vi "statusQuery.vi"(8 "Reply size":i32, 11 "Device ID":i32) -> (0 "statusText":string, 3 "statusCode":i32)   [LabVIEW 2011]
panel:
  out "cyclic status":bool
  out "ramp status":bool
  out "ramp status 2":bool
  out "Reply":string
  out "frameStatus 2":bool
  out "unsigned byte array":u8[](array[numeric])
  out "1 min":u8
  out "1 max":u8
  out "2 min":u8
  out "2 max":u8
  out "frameStatus":bool
  out "Boolean array":bool[](array[boolean])
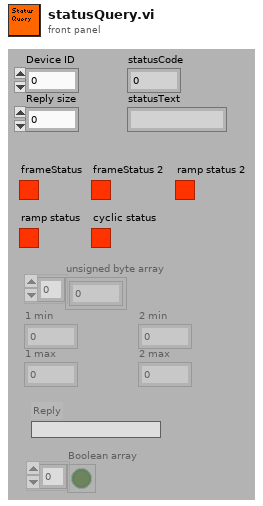
[diagram p1: front panel]
types:
  T1 = cluster{"unsigned byte array[0]":u8, "unsigned byte array[1]":u8, "unsigned byte array[2]":u8, "unsigned byte array[3]":u8, "unsigned byte array[4]":u8, "unsigned byte array[5]":u8, "unsigned byte array[6]":u8, "unsigned byte array[7]":u8, "unsigned byte array[8]":u8}
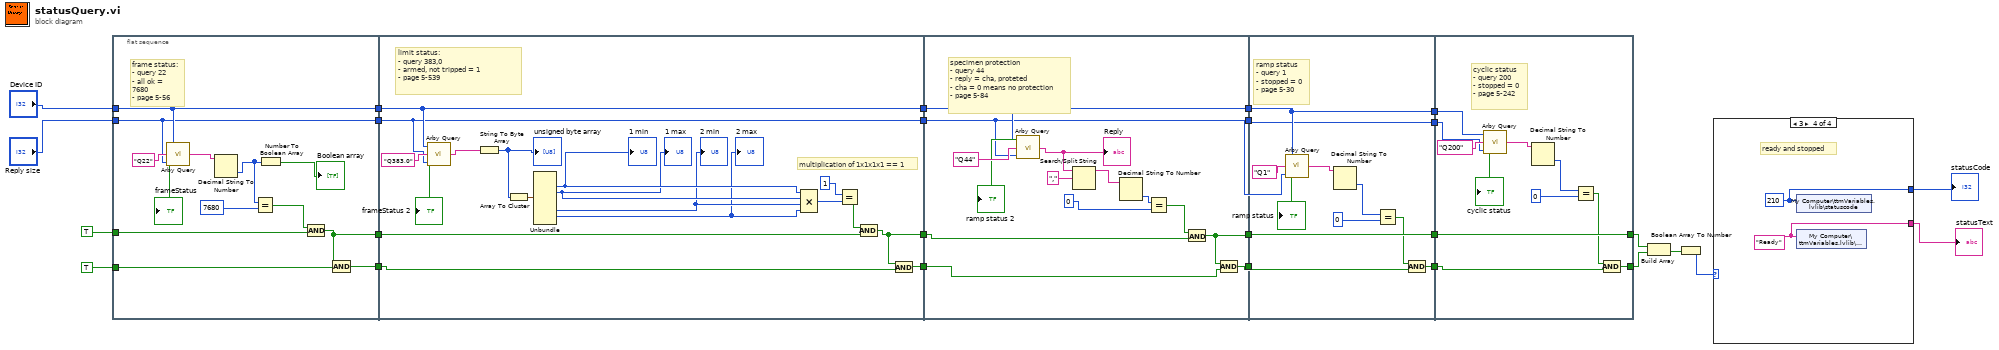
[diagram p0: block diagram]
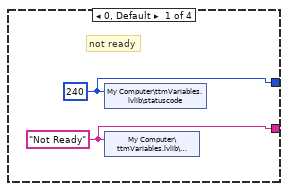
[diagram p2: hidden frame]
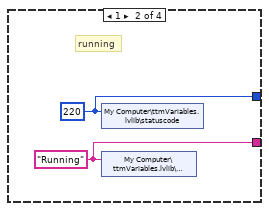
[diagram p3: hidden frame]
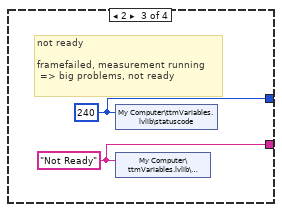
[diagram p4: hidden frame]
diagram:
  n1 = flat-sequence {
    tunnel: "Reply size" -> [w27]
    tunnel: "Device ID" -> [w28]
    tunnel: TRUE -> [w32]
    tunnel: TRUE -> [w30]
    tunnel: [w31] -> w26
    tunnel: [w29] -> w25
    tunnel: [w28] -> w24
    tunnel: [w27] -> w23
    tunnel: w26 -> [w43]
    tunnel: [w40] -> w22
    tunnel: w25 -> [w41]
    tunnel: [w42] -> w21
    tunnel: w24 -> [w55]
    tunnel: [w55] -> w20
    tunnel: w23 -> [w54]
    tunnel: [w54] -> w19
    tunnel: w22 -> [w61]
    tunnel: [w59] -> w18
    tunnel: w21 -> [w60]
    tunnel: [w58] -> w17
    tunnel: w20 -> [w69]
    tunnel: [w69] -> w16
    tunnel: w19 -> [w68]
    tunnel: [w68] -> w15
    tunnel: w18 -> [w82]
    tunnel: w17 -> [w76]
    tunnel: w16 -> [w73]
    tunnel: w15 -> [w72]
    tunnel: [w82] -> w14
    tunnel: [w74] -> w13
    tunnel: [w73] -> w12
    tunnel: [w72] -> w11
    tunnel: [w93] -> w10
    tunnel: w14 -> [w93]
    tunnel: w13 -> [w85]
    tunnel: w12 -> [w87]
    tunnel: w11 -> [w86]
    tunnel: [w83] -> w9
    frame #0 {
      # "frame status:\n- query 22\n- all ok = 7680\n- page 5-56"
      n2 = call "Arby Query.vi"("Reply size"=w27, "Query"="Q22", "Device"=w28) -> ("Reply"=w35:string, "Success"=→"frameStatus":bool)  [unwired: 1 out]
      n3 = Decimal String To Number(string=w35) -> (number=w38:i32)  [unwired: 2 in, 1 out]
      n4 = Equal?(x=w38, y=7680 ("number")) -> (x = y?=w33:bool)
      n5 = Number To Boolean Array(number=w38) -> (Boolean array=→"Boolean array":bool[])
      n6 = Compound Arithmetic op=AND(w33, w32) -> (w31:bool)
      n7 = Compound Arithmetic op=AND(w31, w30) -> (w29:bool)
    }
    frame #1 {
      # "multiplication of 1x1x1x1 == 1"
      # "limit status:\n- query 383,0\n- armed, not tripped = 1\n- page 5-539"
      n8 = call "Arby Query.vi"("Reply size"=w54, "Query"="Q383,0", "Device"=w55) -> ("Reply"=w53:string, "Success"=→"frameStatus 2":bool)  [unwired: 1 out]
      n9 = String To Byte Array(string=w53) -> (unsigned byte array=w52:u8[])
      "unsigned byte array" <- w52
      n10 = Array To Cluster(array=w52) -> (cluster=w51:T1)
      n11 = Unbundle(w51) -> ("unsigned byte array[2]"=w50:u8, "unsigned byte array[3]"=w49:u8, "unsigned byte array[6]"=w48:u8, "unsigned byte array[7]"=w47:u8)  [unwired: 5 out]
      "1 min" <- w50
      "1 max" <- w49
      "2 min" <- w48
      "2 max" <- w47
      n12 = Compound Arithmetic op=MULTIPLY(w50, w49, w48, w47) -> (w46:u8)
      n13 = Equal?(x=u8 1, y=w46) -> (x = y?=w44:bool)
      n14 = Compound Arithmetic op=AND(w44, w43) -> (w40:bool)
      n15 = Compound Arithmetic op=AND(w40, w41) -> (w42:bool)
    }
    frame #2 {
      # "specimen protection\n- query 44\n- reply = cha, proteted\n- cha = 0 means no protection\n- page 5-84"
      n16 = call "Arby Query.vi"("Reply size"=w68, "Query"="Q44", "Device"=w69) -> ("Reply"=w67:string, "Success"=→"ramp status 2":bool)  [unwired: 1 out]
      "Reply" <- w67
      n17 = Search/Split String(string=w67, search string/char (-)=",") -> (substring before match=w65:string)  [unwired: 1 in, 2 out]
      n18 = Decimal String To Number(string=w65) -> (number=w64:i32)  [unwired: 2 in, 1 out]
      n19 = Equal?(x=w64, y=0 ("number")) -> (x = y?=w62:bool)
      n20 = Compound Arithmetic op=AND(w62, w61) -> (w59:bool)
      n21 = Compound Arithmetic op=AND(w59, w60) -> (w58:bool)
    }
    frame #3 {
      # "ramp status\n- query 1\n- stopped = 0\n- page 5-30"
      n22 = call "Arby Query.vi"("Reply size"=w72, "Query"="Q1", "Device"=w73) -> ("Reply"=w79:string, "Success"=→"ramp status":bool)  [unwired: 1 out]
      n23 = Decimal String To Number(string=w79) -> (number=w78:i32)  [unwired: 2 in, 1 out]
      n24 = Equal?(x=w78, y=0 ("number")) -> (x = y?=w75:bool)
      n25 = Compound Arithmetic op=AND(w75, w76) -> (w74:bool)
    }
    frame #4 {
      # "cyclic status\n- query 200\n- stopped = 0\n- page 5-242"
      n26 = call "Arby Query.vi"("Reply size"=w86, "Query"="Q200", "Device"=w87) -> ("Reply"=w90:string, "Success"=→"cyclic status":bool)  [unwired: 1 out]
      n27 = Decimal String To Number(string=w90) -> (number=w89:i32)  [unwired: 2 in, 1 out]
      n28 = Equal?(x=w89, y=0 ("number")) -> (x = y?=w84:bool)
      n29 = Compound Arithmetic op=AND(w84, w85) -> (w83:bool)
    }
  }
  n30 = Build Array(w10, w9) -> (w8:bool[])
  n31 = Boolean Array To Number(Boolean array=w8) -> (number=w7:u32)
  n32 = case shown="3" w7 {
    tunnel: [w95 w97 w99 w101] -> w2
    tunnel: [w94 w96 w98 w100] -> w1
    frame 0, Default {
      w94 = "Not Ready" ("statusText")
      w95 = 240 ("statusCode")
      # "not ready"
      n33 = shared-variable "My Computer\\ttmVariables.lvlib\\statuscode"(w95) -> ()  [unwired: 1 in, 1 out]
      n34 = shared-variable "My Computer\\ttmVariables.lvlib\\statustext"(w94) -> ()  [unwired: 1 in, 1 out]
    }
    frame 1 {
      w96 = "Running" ("statusText")
      w97 = 220 ("statusCode")
      # "running"
      n35 = shared-variable "My Computer\\ttmVariables.lvlib\\statuscode"(w97) -> ()  [unwired: 1 in, 1 out]
      n36 = shared-variable "My Computer\\ttmVariables.lvlib\\statustext"(w96) -> ()  [unwired: 1 in, 1 out]
    }
    frame 2 {
      w98 = "Not Ready" ("statusText")
      w99 = 240 ("statusCode")
      # "not ready\n\nframefailed, measurement running\n => big problems, not ready"
      n37 = shared-variable "My Computer\\ttmVariables.lvlib\\statuscode"(w99) -> ()  [unwired: 1 in, 1 out]
      n38 = shared-variable "My Computer\\ttmVariables.lvlib\\statustext"(w98) -> ()  [unwired: 1 in, 1 out]
    }
    frame 3 {
      w100 = "Ready" ("statusText")
      w101 = 210 ("statusCode")
      # "ready and stopped"
      n39 = shared-variable "My Computer\\ttmVariables.lvlib\\statuscode"(w101) -> ()  [unwired: 1 in, 1 out]
      n40 = shared-variable "My Computer\\ttmVariables.lvlib\\statustext"(w100) -> ()  [unwired: 1 in, 1 out]
    }
  }
  "statusCode" <- w2
  "statusText" <- w1
